vi "Flow device cluster to String.vi"(11 "Heater Device Settings":T1) -> (3 "Data to send":string="EXCT:TYPE:Unipolar:MAG:10.00:EXCT:NICK:MB1.T1:LOOP:AUX:None:PSET:1.0:HTR:None:ISET:1.0:HAUT:Manual:HSET:0.0:PIDT:Manual:DSET:1.0:TSET:0K:LVL:MB1.T1:LOOP:MAN:HVER:0:FVER:20.6:SERL:102750119:MAN:CAL:OFFS:0.0000:COLD:1.0000:INT:Linear:SCAL:1.0000:FILE:RP5.DAT:HOTL:1023.1500:CAL:TYPE:PTC:SIG:VOLT:1405.9mV:CURR:10µA:TEMP:1023.15K:POWR:14.059µW:RES:140590?:SLOP:137.409?/K:FLOW:NOT_FOUND:SIG:TEMP\n")   [LabVIEW 2016, in "Mercury iXX.lvlib" / "Flow.lvlib"]
uses:
  Flow.lvlib
  Controls/Flow Device (Set).ctl
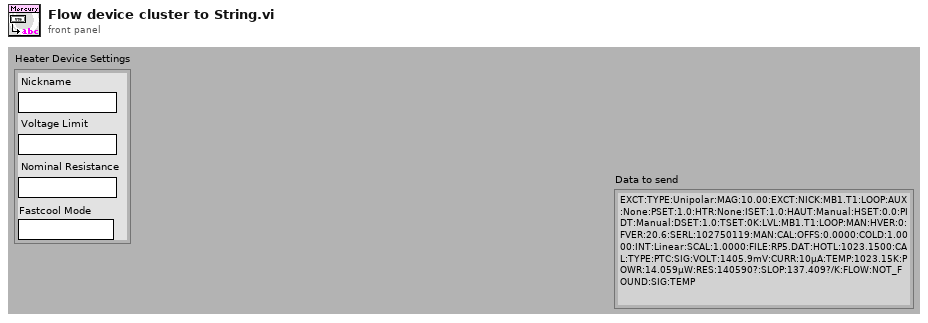
[diagram p1: front panel]
types:
  T1 = typedef "Mercury iXX.lvlib/Flow.lvlib/Flow Device (Set).ctl" = cluster{"Nickname":string, "Voltage Limit":string, "Nominal Resistance":string, "Fastcool Mode":string}
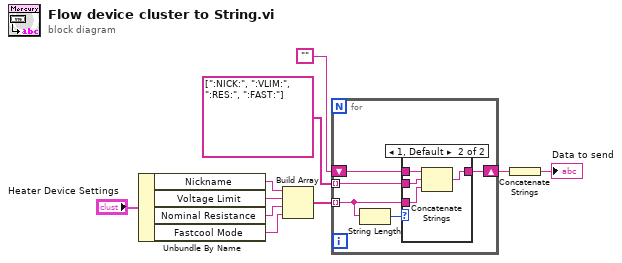
[diagram p0: block diagram]
diagram:
  n1 = Unbundle By Name("Heater Device Settings") -> ("Nickname"=w3:string, "Voltage Limit"=w4:string, "Nominal Resistance"=w9:string, "Fastcool Mode"=w1:string)
  n2 = Build Array(w3, w4, w9, w1) -> (w2:string[])
  n3 = for {
    tunnel: w2 -> [w14] mode=indexing
    tunnel: string[] [":NICK:", ":VLIM:", ":RES:", ":FAST:"] ("Excitation") -> [w13] mode=indexing
    shift-right: [w12] -> w5
    shift-left: "" -> [w11]
    n4 = String Length(string=w14) -> (length=w15:i32)
    n5 = case shown="1, Default" w15 {
      tunnel: w14 -> [_ w19]
      tunnel: [w16 w20] -> w12
      tunnel: w13 -> [_ w18]
      tunnel: w11 -> [w16 w17]
      frame 0 {
      }
      frame 1, Default {
        n6 = Concatenate Strings(w17, w18, w19) -> (w20:string)
      }
    }
  }
  n7 = Concatenate Strings(w5) -> (→"Data to send":string)
